vi "GetInputValues.vi"(0 "handle in":i32, 1 "UnitAddress(0)":u16, 2 "Channel(0)":u8, 3 "ResponseAddress(0)":u8, 5 "error in":errorcluster) -> (14 "handle out":i32, 15 "AnalogueValue (V)":dbl, 16 "RefInput":bool, 17 "AllInputs":T1, 18 "TtlIo1":u8, 19 "error out":errorcluster)   [LabVIEW 2014, in "Sixpack - Driver.lvlib"]
doc: "Die Analogkanäle sind für ratiometrische Messungen von Widerstandsteilern ausgelegt. Kanal 0 bis 5 bezeichnen die Eingänge an den Motorsteckern (A_In), Kanal 6 ist der externe Eingang, Kanal 7 misst die Versorgungsspannung des PACKs (1V ergibt Wert 22). Die Referenzeingänge (RefIn) geben den anliegenden Pegel invertiert aus. Die Variable AllInputs enthält die Werte aller digitalen Eingänge. Die Bits 0-5 enthalten die invertierten Pegel der Referenzeingänge (RefIn), Bit 6 und 7 geben die Jumperkonfiguration für die CAN Adressierung zurück (siehe auch Kapitel 3.1.2)."
uses:
  Sixpack - Driver.lvlib
  DLL/PackDLL.dll
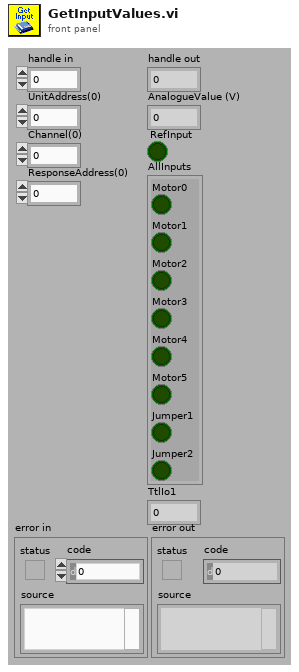
[diagram p1: front panel]
types:
  T1 = cluster{"Motor0":bool, "Motor1":bool, "Motor2":bool, "Motor3":bool, "Motor4":bool, "Motor5":bool, "Jumper1":bool, "Jumper2":bool}
  T2 = cluster{"Boolean array[0]":bool, "Boolean array[1]":bool, "Boolean array[2]":bool, "Boolean array[3]":bool, "Boolean array[4]":bool, "Boolean array[5]":bool, "Boolean array[6]":bool, "Boolean array[7]":bool}
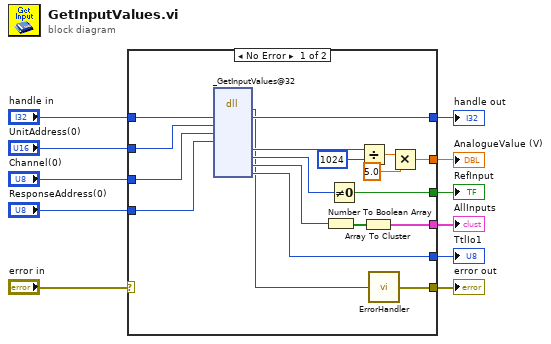
[diagram p0: block diagram]
diagram:
  n1 = case shown="No Error" "error in" {
    selector: "error in" -> [_ w31]
    tunnel: "handle in" -> [w29 w30]
    tunnel: "UnitAddress(0)" -> [w28 _]
    tunnel: "Channel(0)" -> [w27 _]
    tunnel: [w24 _] -> w8
    tunnel: [w23 _] -> w7
    tunnel: [w21 _] -> w6
    tunnel: "ResponseAddress(0)" -> [w20 _]
    tunnel: [w17 _] -> w4
    tunnel: [w14 w30] -> w3
    tunnel: [w13 w31] -> w2
    frame No Error {
      n2 = dll-call lib="D:/CS-Source/LV2014/GPL/instr.lib/SixPack/PackDLL/DLL/PackDLL.dll" fn="_GetInputValues@32" label="GetInputValues"("HANDLE"=w29, "UnitAddress"=w28, "Channel"=w27, "ResponseAddress"=w20) -> ("BOOLEAN"=w12:i8, "HANDLE"=w14:i32, "AnalogueValue"=w15:u16, "RefInput"=w19:u8, "AllInputs"=w18:u8, "TtlIo1"=w17:u8)  [unwired: 10 in, 2 out]
      n3 = Number To Boolean Array(number=w18) -> (Boolean array=w22:bool[])
      n4 = Not Equal To 0?(x=w19) -> (x != 0?=w23:bool)
      n5 = Divide(x=w15, y=u16 1024) -> (x/y=w26:dbl)
      n6 = Array To Cluster(array=w22) -> (cluster=w21:T2)
      n7 = call "ErrorHandler.vi"("BOOLEAN"=w12) -> ("error out"=w13:errorcluster)
      n8 = Multiply(x=w26, y=5.0) -> (x*y=w24:dbl)
    }
    frame Error {
    }
  }
  "handle out" <- w3
  "AnalogueValue (V)" <- w8
  "RefInput" <- w7
  "TtlIo1" <- w4
  "AllInputs" <- w6
  "error out" <- w2
